vi "BoxSetCommandReady.vi"() -> (0 "BoxCommandReady":bool)   [LabVIEW 2023]
uses:
  BoxGlobals.vi
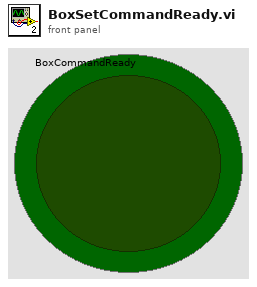
[diagram p1: front panel]
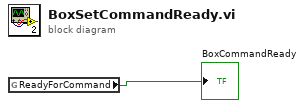
[diagram p0: block diagram]
diagram:
  n1 = global read "BoxGlobals.vi" "ReadyForCommand"() -> (→"BoxCommandReady":bool)
